vi "Continuous Swept-Sine Measurements.vi"() -> ()   [LabVIEW 2018]
doc: "Overview:\nThis VI demonstrates simultaneous frequency response, level, and distortion measurements using a discrete swept-sine technique. This example implements analog input and analog output with 'Finite Samples' sample mode which minimizes sensitivity to bandwidth issues that can cause run-time errors when performing continuous measurements. This VI also demonstrates how finite acquisitions can be read in a single large block or in a series of smaller reads.\n\nRequirements:\nLabVIEW Full Development System\nSound and Vibration Toolkit\n\nInstructions:\n1. Connect the DUT to the DSA device.\n2. Select the AO excitation channel, AI stimulus channel, and AI response channel.\n3. Run the VI.\n\nDetails:\nThis VI performs a swept sine measurement to obtain the root-mean-square (RMS) levels of the acquired stimulus and response, the frequency response of the device under test (DUT), and the harmonic distortion on the response channel. You specify the source and measurement parameters, and the swept sine VIs handle all the DAQ-specific controls required to perform the measurement. You have direct control over the source, input, averaging, and display parameters. You also specify the engineering units to use for the swept sine measurements.\n\nYou can view the time records of the acquired stimulus and response signals. From these graphs, you can see that the transition to the next test frequency always occurs at a zero crossing to minimize non-linear disturbances to the DUT. The RMS levels, frequency response, and harmonic distortion are shown on different tabs."
uses:
  <vilib>/sound2/lvsound2.llb/Sampling Mode.ctl
  <vilib>/sound2/lvsound2.llb/Sound Data Format.ctl
  <vilib>/addons/_NISVFA/_Shared subVIs/Controls/svc_Window.ctl
  <vilib>/addons/_NISVFA/_Generation/Signal Generation/SV Signal/SV Signal.lvclass/SV Signal.ctl
  <vilib>/addons/_NISVFA/_Shared subVIs/Common/svc_Get Waveform Subset (Index).vi
  <vilib>/addons/_NISVFA/_Generation/Signal Generation/SV Signal/Write Leading Synchronization Pulse Enable.vi
  <vilib>/addons/_NISVFA/_Generation/Signal Generation/SV Signal/Write Ramp-Up.vi
  <vilib>/addons/_NISVFA/_Generation/Signal Generation/SV Signal/Write Ramp-Down.vi
  <vilib>/addons/_NISVFA/_Shared subVIs/Common/svc_Get Array Subset (Index).vi
  <vilib>/addons/_NISVFA/_Shared subVIs/Common/svc_Coerce Index and Length.vi
  <vilib>/addons/_NISVFA/_Shared subVIs/Common/svc_Conditional Merge Error.vi
  <vilib>/addons/_NISVFA/_Generation/Signal Generation/SV Continuous Sweep/SV Continuous Sweep.lvclass
  C:/Program Files (x86)/National Instruments/LabVIEW 2018/vi.lib/addons/_NISVFA/_Generation/Signal Generation/SV Signal/SV Signal.lvclass
  <vilib>/addons/_NISVFA/_Generation/Signal Generation/SV Continuous Sweep/Configure Continuous Sweep.vi
  <vilib>/addons/_NISVFA/_Generation/Signal Generation/SV Signal/Write Ramp Parameters.vi
  <vilib>/addons/_NISVFA/_Generation/Signal Generation/SV Signal/Write DC Offset.vi
  <vilib>/addons/_NISVFA/_Generation/Signal Generation/SV Signal/Write Transition Profile.vi
  <vilib>/addons/_NISVFA/_Generation/Signal Generation/SV Signal/Write Pre-Measurement Settling Duration.vi
  <vilib>/addons/_NISVFA/_Generation/Signal Generation/SV Signal/Write Post-Measurement Settling Duration.vi
  <vilib>/sound2/lvsound2.llb/Sound Output Set Volume (Single).vi
  <vilib>/sound2/lvsound2.llb/Sound Output Write (DBL Single).vi
  <vilib>/sound2/lvsound2.llb/Sound Input Read (DBL).vi
  <vilib>/addons/_NISVFA/_Baseband FFT/SVFA FFT Spectrum (Complex) (1 Ch).vi
  <vilib>/addons/Sound and Vibration/svt_Single Tone Measurements/SVT Gain and Phase (Frequency).vi
  <vilib>/addons/Sound and Vibration/svt_Distortion/SVT THD and Harmonic Components (Frequency) (1 Ch).vi
  <vilib>/addons/_NISVFA/_Generation/Signal Generation/SV Signal/SV Signal.lvclass
  Program Files (x86)/National Instruments/LabVIEW 2018/examples/Sound and Vibration/SoundVib_Audio Examples.lvlib
  <vilib>/addons/Sound and Vibration/svt_Continuous Swept Sine/SoundVib_ContSweptSine.lvlib
  <vilib>/addons/Sound and Vibration/svt_Distortion/SoundVib_Distortion.lvlib
  <vilib>/addons/Sound and Vibration/svt_Single Tone Measurements/SoundVib_SingleTone.lvlib
panel:
  in  "device In":u32
  in  "device Out":u32=1
  out "Magnitude":cluster{"frequency":dbl[], "magnitude":dbl[]}(graph)
  out "Phase":cluster{"frequency":dbl[], "magnitude":dbl[]}(graph)
  out "THD":cluster{"frequency":dbl[], "THD":dbl[]}(graph)
  in  "Samples/Sec":dbl=44100.0
  in  "DC offset":dbl format="%.2f V"
  in  "amplitude":dbl=1.0 format="%.2p V"
  in  "frequency range":cluster{"start":dbl, "stop":dbl}={"start"=20000.0, "stop"=40.0} {"stop" min=0.0 format="%.2f Hz"; "start" min=0.0 format="%.2f Hz"}
  in  "duration":dbl=3.0 min=0.0 format="%.2f s"
  out "test time":u32 format="%.0f ms"
  out "error Mic":errorcluster
  out "error Spkr":errorcluster
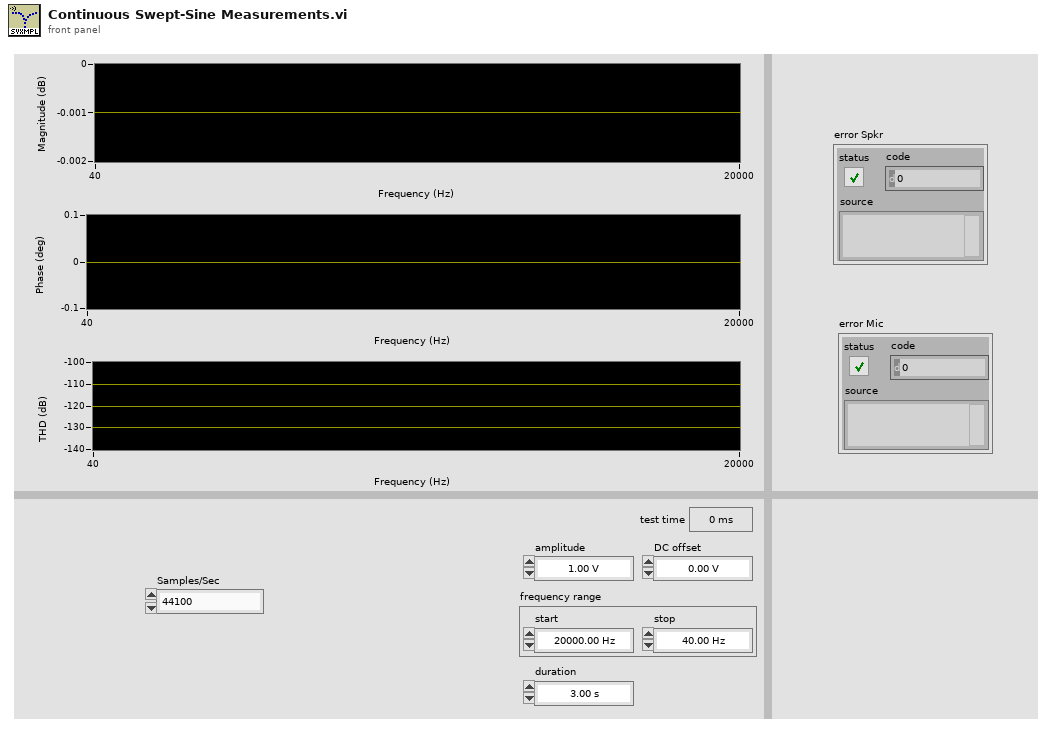
[diagram p1: front panel]
types:
  T1 = typedef "Sound Data Format.ctl" = cluster{"sample rate (S/s)":dbl, "number of channels":i32, "bits per sample":i32}
  T2 = typedef "Sampling Mode.ctl" = i32
  T3 = cluster{"start frequency":dbl, "stop frequency":dbl, "number of steps":i32}
  T4 = cluster{"profile":enum16{"Linear", "Half cosine"}, "durations [s]":cluster{"ramp-up":dbl, "transition":dbl, "ramp-down":dbl}}
  T5 = typedef "Sound Output Task ID.ctl" = u32
  T6 = typedef "Sound Input Task ID.ctl" = u32
  T7 = cluster{"averaging mode":enum16{"No averaging", "Vector averaging", "RMS averaging", "Peak hold"}, "weighting mode":enum16{"Linear", "Exponential"}, "number of averages":u32, "linear mode":enum16{"One shot", "Auto restart"}}
  T8 = typedef "svc_Window.ctl" = u32
  T9 = typedef "svc_Spectrum Info.ctl" = cluster{"channel name":string, "description":string, "x-axis units":T10, "spectral info":cluster{"spectrum type":T11, "linear/dB":enum16{"linear", "dB"}, "window":u16, "window size":i32, "FFT size":i32}, "engineering units":T12, "custom label":string, "dB reference [EU]":dbl, "peak units":enum16{"rms", "peak", "peak-peak"}, "weighting filter":T13, "spectral density?":bool, "unit label":string, "spectrum skewed?":bool, "complimentary spectrum units":T14}
  T10 = typedef "svc_X-Axis Units.ctl" = u16
  T11 = typedef "svc_Spectrum Type.ctl" = enum16{"FFT Spectrum [complex]", "Amplitude [Magnitude]", "Power [Magnitude^2]", "Cross Spectrum [complex]", "Frequency Response [Complex]"}
  T12 = typedef "svc_Engineering Units Text Ring.ctl" = u16
  T13 = typedef "svc_Weighting Filter Text Ring.ctl" = u16
  T14 = typedef "svc_Complimentary Spectrum Units.ctl" = enum16{"none", "radians", "degrees", "cycles", "imaginary"}
  T15 = cluster{"complex spectrum response":cluster{"f0":dbl, "df":dbl, "complex spectrum":cdb[]}, "spectrum info":T9}
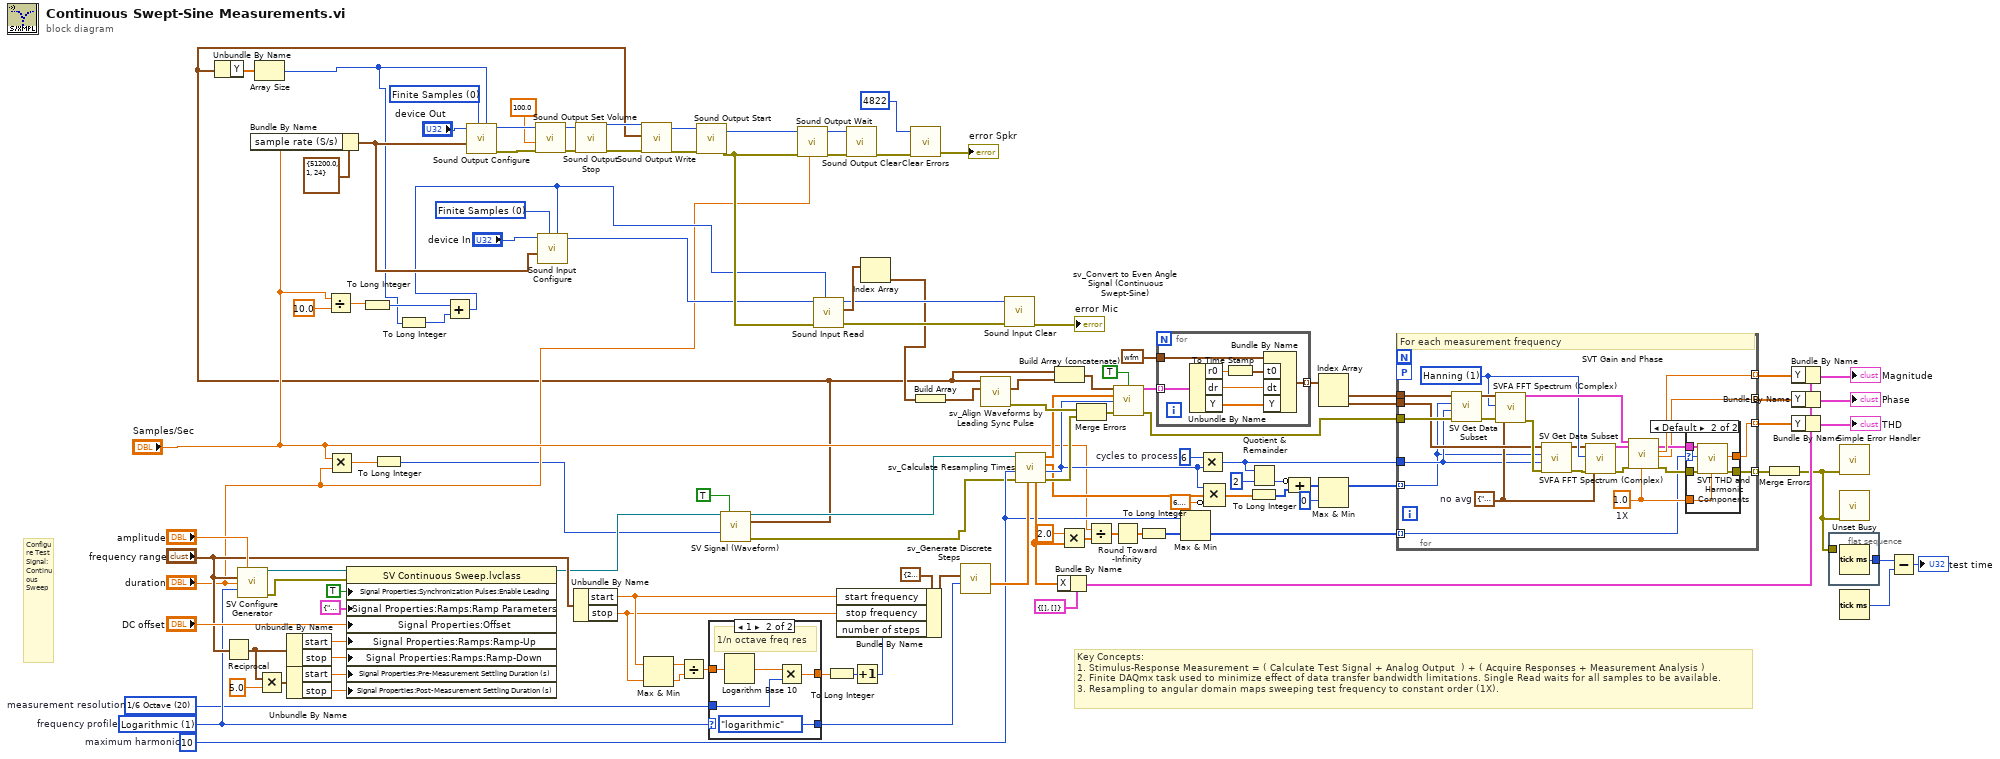
[diagram p0: block diagram]
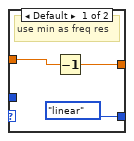
[diagram p2: hidden frame]
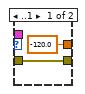
[diagram p3: hidden frame]
diagram:
  w40 = T2 0 items=["Finite Samples", "Continuous Samples"] ("sample mode")
  w42 = T2 0 items=["Finite Samples", "Continuous Samples"] ("sample mode")
  w49 = u16 20 items=["1/3 Octave"=10, "1/6 Octave"=20, "1/12 Octave"=40, "1/24 Octave"=80, "1/48 Octave"=160]  # measurement resolution
  w64 = u16 1 items=["Linear", "Logarithmic"]  # frequency profile
  w91 = 6  # cycles to process
  w52 = 10  # maximum harmonic
  # "Key Concepts:\n1. Stimulus-Response Measurement = ( Calculate Test Signal + Analog Output  ) + ( Acquire Responses + Measurement Analysis )\n2. Finite DAQmx task used to minimize effect of data transfer bandwidth limitations. Single Read waits for all samples to be available.\n3. Resampling to angular domain maps sweeping test frequency to constant order (1X)."
  # "Configure Test Signal: \nContinuous Sweep"
  n1 = Reciprocal(x="frequency range") -> (1/x=w79:cluster{"start":dbl, "stop":dbl})
  n2 = call-poly <vilib>:"SV Configure Generator.vi"("amplitude"="amplitude", "frequency range [Hz]"="frequency range", "duration [s]"="duration", "profile"=w64) -> ("signal configuration"=w119:refnum<class "SV Continuous Sweep.lvclass">, "error out"=w116:errorcluster)  [unwired: 10 in]
  n3 = Bundle By Name(cluster=T1 {"sample rate (S/s)"=51200.0, "number of channels"=1, "bits per sample"=24} ("sound format"), "sample rate (S/s)"="Samples/Sec") -> (w34:T1)
  n4 = Multiply(x=w79, y=5.0 ("stop")) -> (x*y=w80:cluster{"start":dbl, "stop":dbl})
  n5 = Unbundle By Name(w79) -> ("start"=w78:dbl, "stop"=w77:dbl)
  n6 = Unbundle By Name(w80) -> ("start"=w81:dbl, "stop"=w82:dbl)
  n7 = Divide(x="Samples/Sec", y=10.0) -> (x/y=w31:dbl)
  n8 = Multiply(x="Samples/Sec", y="duration") -> (x*y=w8:dbl)
  n9 = property class="SV Continuous Sweep.lvclass"(reference=w119, error in=w116, "Signal Properties:Synchronization Pulses:Enable Leading"=TRUE ("Synchronization Pulses:Enable Leading"), "Signal Properties:Ramps:Ramp Parameters"=T4 {"profile"=enum."Half cosine", "durations [s]"={"ramp-up"=0.01, "transition"=0.0, "ramp-down"=0.01}} ("Ramp Parameters"), "Signal Properties:Offset"="DC offset", "Signal Properties:Ramps:Ramp-Up"=w78, "Signal Properties:Ramps:Ramp-Down"=w77, "Signal Properties:Pre-Measurement Settling Duration (s)"=w81, "Signal Properties:Post-Measurement Settling Duration (s)"=w82) -> (reference out=w11:refnum<class "SV Continuous Sweep.lvclass">)  [unwired: 1 out]
  n10 = To Long Integer(number=w31) -> (32bit integer=w30:i32)
  n11 = To Long Integer(number=w8) -> (32bit integer=w7:i32)
  n12 = Unbundle By Name("frequency range") -> ("start"=w68:dbl, "stop"=w67:dbl)
  n13 = Max & Min(x=w68, y=w67) -> (max(x,y)=w73:dbl, min(x,y)=w72:dbl)
  n14 = Divide(x=w73, y=w72) -> (x/y=w71:dbl)
  n15 = case shown="1" w64 {
    tunnel: w71 -> [w121 w127]
    tunnel: [w120 w125] -> w70
    tunnel: [enum16{"linear", "logarithmic"}."linear" ("spacing") enum16{"linear", "logarithmic"}."logarithmic" ("spacing")] -> w65
    tunnel: w49 -> [_ w123]
    frame Default {
      # "use min as freq res"
      n16 = Decrement(x=w121) -> (x-1=w120:dbl)
    }
    frame 1 {
      # "1/n octave freq res"
      n17 = Logarithm Base 10(1:w127) -> (0:w126:dbl)
      n18 = Multiply(x=w126, y=w123) -> (x*y=w125:dbl)
    }
  }
  n19 = call-dynamic "SV Signal (Waveform).vi"("signal configuration"=w11, "reset"=TRUE, "samples"=w7) -> ("signal configuration"=w5:refnum<class "SV Continuous Sweep.lvclass">, "output waveform"=w3:waveform(dbl), "error out"=w4:errorcluster)  [unwired: 7 in, 3 out]
  n20 = Unbundle By Name(w3) -> ("Y"=w33:dbl[])
  n21 = Array Size(array=w33) -> (size(s)=w28:i32)
  n22 = To Long Integer(number=w28) -> (32bit integer=w29:i32)
  n23 = Add(x=w30, y=w29) -> (x+y=w18:i32)
  n24 = call <vilib>:"Sound Output Configure.vi"("number of samples/ch"=w28, "sample mode"=w42, "sound format"=w34, "device ID"="device Out") -> ("error out"=w46:errorcluster, "task ID"=w45:T5)  [unwired: 6 in]
  n25 = call-poly <vilib>:"Sound Output Set Volume.vi"("error in (no error)"=w46, "volume"=100.0, "task ID"=w45) -> ("error out"=w38:errorcluster, "task ID out"=w39:T5)  [unwired: 7 in]
  n26 = call <vilib>:"Sound Input Configure.vi"("number of samples/ch"=w18, "sample mode"=w40, "sound format"=w34, "device ID"="device In") -> ("task ID"=w17:T6)  [unwired: 6 in, 1 out]
  n27 = call <vilib>:"Sound Output Stop.vi"("error in (no error)"=w38, "task ID"=w39) -> ("error out"=w36:errorcluster, "task ID out"=w37:T5)  [unwired: 8 in]
  n28 = call-poly <vilib>:"Sound Output Write.vi"("error in (no error)"=w36, "data"=w3, "task ID"=w37) -> ("error out"=w19:errorcluster, "task ID out"=w20:T5)  [unwired: 7 in]
  n29 = call <vilib>:"Sound Output Start.vi"("error in (no error)"=w19, "task ID"=w20) -> ("error out"=w24:errorcluster, "task ID out"=w25:T5)  [unwired: 8 in]
  n30 = call <vilib>:"Sound Output Wait.vi"("timeout (sec)"="duration", "error in (no error)"=w24, "task ID"=w25) -> ("error out"=w27:errorcluster, "task ID out"=w26:T5)  [unwired: 7 in]
  n31 = call-poly <vilib>:"Sound Input Read.vi"("number of samples/ch"=w18, "error in (no error)"=w24, "task ID"=w17) -> ("error out"=w15:errorcluster, "data"=w23:waveform(dbl)[], "task ID out"=w16:T6)  [unwired: 6 in]
  n32 = To Long Integer(number=w70) -> (32bit integer=w69:i32)
  n33 = call <vilib>:"Sound Output Clear.vi"("error in (no error)"=w27, "task ID"=w26) -> ("error out"=w22:errorcluster)  [unwired: 9 in]
  n34 = Increment(x=w69) -> (x+1=w66:i32)
  n35 = Bundle By Name(cluster=T3 {"start frequency"=20.0, "stop frequency"=20000.0, "number of steps"=100} ("sweep frequencies"), "start frequency"=w68, "stop frequency"=w67, "number of steps"=w66) -> (w74:T3)
  n36 = Index Array(array=w23) -> (element=w14:waveform(dbl))  [unwired: 1 in]
  n37 = call <vilib>:"Clear Errors.vi"("error in (no error)"=w22, "specific error code to clear (0: all)"=4822) -> ("error out"=→"error Spkr":errorcluster)  [unwired: 4 in, 1 out]
  n38 = Build Array(w14) -> (w47:waveform(dbl)[])
  n39 = call <vilib>:"sv_Generate Discrete Steps.vi"("spacing"=w65, "steps"=w74) -> ("frequency list"=w60:dbl[])  [unwired: 8 in, 1 out]
  n40 = call "sv_Align Waveforms by Leading Sync Pulse.vi"("response signals"=w47, "alignment reference signal"=w3) -> ("error out"=w101:errorcluster, "aligned signals"=w2:waveform(dbl)[])  [unwired: 5 in, 3 out]
  n41 = call <vilib>:"Sound Input Clear.vi"("error in (no error)"=w15, "task ID"=w16) -> ("error out"=→"error Mic":errorcluster)  [unwired: 9 in]
  n42 = call "sv_Calculate Resampling Times.vi"("measurement frequencies in (Hz)"=w60, "error in"=w4, "maximum harmonic"=w52, "continuous sweep configuration"=w5) -> ("error out"=w100:errorcluster, "samples/rev"=w90:i32, "measurement phases (rad)"=w61:dbl[], "resampling times (s)"=w62:dbl[], "measurement frequencies (Hz)"=w53:dbl[])  [unwired: 1 in, 2 out]
  n43 = Build Array (concatenate)(w3, w2) -> (w1:waveform(dbl)[])
  n44 = Bundle By Name(cluster=cluster{"X":dbl[], "Y":dbl[]} {"X"=[], "Y"=[]} ("THD vs Amplitude"), "X"=w53) -> (w109:cluster{"X":dbl[], "Y":dbl[]})
  n45 = Multiply(x=2.0 ("y"), y=w53) -> (x*y=w57:dbl[])
  n46 = Merge Errors(w101, w100) -> (w99:errorcluster)
  n47 = Divide(x="Samples/Sec", y=w57) -> (x/y=w56:dbl[])
  n48 = Round Toward -Infinity(1:w56) -> (0:w55:dbl[])
  n49 = call <vilib>:"sv_Convert to Even Angle Signal (Continuous Swept-Sine).vi"("scaled signals [EU]"=w1, "reset? (F)"=TRUE, "new sample time [s]"=w62, "new samples/rev"=w90, "error in (no error)"=w99) -> ("even-angle signals"=w105:cluster{"r0":dbl, "dr":dbl, "Y":dbl[]}[], "error out"=w48:errorcluster)  [unwired: 6 in, 3 out]
  n50 = To Long Integer(number=w55) -> (32bit integer=w51:i32[])
  n51 = for {
    tunnel: w105 -> [w134] mode=indexing
    tunnel: waveform(dbl) {"t0"=timestamp(0 s since 1904-01-01), "dt"=1.0, "Y"=[]} ("waveform out") -> [w129]
    tunnel: [w128] -> w103 mode=indexing
    n52 = Unbundle By Name(w134) -> ("r0"=w133:dbl, "dr"=w131:dbl, "Y"=w130:dbl[])
    n53 = To Time Stamp(1:w133) -> (0:w132:timestamp)
    n54 = Bundle By Name(cluster=w129, "t0"=w132, "dt"=w131, "Y"=w130) -> (w128:waveform(dbl))
  }
  n55 = Max & Min(x=w52, y=w51) -> (min(x,y)=w50:i32[])  [unwired: 1 out]
  n56 = Multiply(x=w91, y=w90) -> (x*y=w88:i32)
  n57 = Compound Arithmetic op=MULTIPLY(w90, w61, invert 6.283185307179586) -> (w59:dbl[])
  n58 = To Long Integer(number=w59) -> (32bit integer=w87:i32[])
  n59 = Quotient & Remainder(x=w88, y=2 ("x")) -> (floor(x/y)=w89:i32)  [unwired: 1 out]
  n60 = Compound Arithmetic op=ADD(invert w89, w87) -> (w85:i32[])
  n61 = Index Array(array=w103) -> (element #1=w97:waveform(dbl), element #2=w96:waveform(dbl))  [unwired: 2 in]
  n62 = Max & Min(x=w85, y=0 ("x")) -> (max(x,y)=w84:i32[])  [unwired: 1 out]
  n63 = for {
    tunnel: w48 -> [w157]
    tunnel: [w151] -> w98 mode=indexing
    tunnel: [w150] -> w95 mode=indexing
    tunnel: w97 -> [w149]
    tunnel: w96 -> [w148]
    tunnel: [w140] -> w93 mode=indexing
    tunnel: [w139] -> w94 mode=indexing
    tunnel: w88 -> [w138]
    tunnel: w84 -> [w137] mode=indexing
    tunnel: w50 -> [w135] mode=indexing
    workers-P: _ -> [_]
    w136 = 1.0  # 1X
    w141 = T7 {"averaging mode"=enum."No averaging", "weighting mode"=enum."Exponential", "number of averages"=10, "linear mode"=enum."One shot"}  # no avg
    w152 = T8 1 items=["None"=0, "Hanning"=1, "Hamming"=2, "Blackman-Harris"=3, "Exact Blackman"=4, "Blackman"=5, "Flat Top"=6, "4 Term B-Harris "=7, "7 Term B-Harris"=8, "Low Sidelobe"=9, "Force"=64, "Exponential"=65, "Blackman Nuttall"=11, "Triangle"=30, "Bartlett-Hanning"=31, "Bohman"=32, "Parzen"=33, "Welch"=34, "Kaiser"=60, "Dolph-Chebyshev"=61, "Gaussian"=62] ("window")
    # "For each measurement frequency"
    n64 = call-poly <vilib>:"SV Get Data Subset.vi"("error in (no error)"=w157, "length (-1 = all)"=w138, "start index (0)"=w137, "waveform in"=w149) -> ("error out"=w155:errorcluster, "waveform subset"=w156:waveform(dbl))  [unwired: 2 in, 4 out]
    n65 = call-poly <vilib>:"SVFA FFT Spectrum (Complex).vi"("scaled signal [EU]"=w156, "window"=w152, "error in"=w155, "averaging parameters"=w141) -> ("complex spectrum"=w153:T15, "error out"=w154:errorcluster)  [unwired: 12 in, 2 out]
    n66 = call-poly <vilib>:"SV Get Data Subset.vi"("error in (no error)"=w154, "length (-1 = all)"=w138, "start index (0)"=w137, "waveform in"=w148) -> ("error out"=w146:errorcluster, "waveform subset"=w147:waveform(dbl))  [unwired: 2 in, 4 out]
    n67 = call-poly <vilib>:"SVFA FFT Spectrum (Complex).vi"("scaled signal [EU]"=w147, "window"=w152, "error in"=w146, "averaging parameters"=w141) -> ("complex spectrum"=w143:T15, "error out"=w142:errorcluster)  [unwired: 12 in, 2 out]
    n68 = call-poly <vilib>:"SVT Gain and Phase.vi"("complex spectrum\nstimulus X"=w153, "complex spectrum\nresponse Y"=w143, "error in (no error)"=w142, "expected fundamental frequency [Hz]"=w136) -> ("dup complex spectrum\nresponse Y"=w145:T15, "gain"=w150:dbl, "phase lag"=w139:dbl, "error out"=w144:errorcluster)  [unwired: 8 in, 4 out]
    n69 = case shown="Default" w135 {
      selector: w135 -> [_ w160]
      tunnel: [w159 w165] -> w151
      tunnel: w145 -> [_ w164]
      tunnel: w144 -> [w159 w163]
      tunnel: [-120.0 ("THD") w162] -> w140
      tunnel: w136 -> [_ w161]
      frame ..1 {
      }
      frame Default {
        n70 = call-poly <vilib>:"SVT THD and Harmonic Components.vi"("complex spectrum"=w164, "maximum harmonic"=w160, "error in (no error)"=w163, "expected fundamental frequency [Hz]"=w161) -> ("THD"=w162:dbl, "error out"=w165:errorcluster)  [unwired: 8 in, 6 out]
      }
    }
  }
  n71 = Merge Errors(w98) -> (w63:errorcluster)
  n72 = Bundle By Name(cluster=w109, "Y"=w95) -> (→"Magnitude":cluster{"X":dbl[], "Y":dbl[]})
  n73 = Bundle By Name(cluster=w109, "Y"=w94) -> (→"Phase":cluster{"X":dbl[], "Y":dbl[]})
  n74 = Bundle By Name(cluster=w109, "Y"=w93) -> (→"THD":cluster{"X":dbl[], "Y":dbl[]})
  n75 = flat-sequence {
    tunnel: [w166] -> w108
    tunnel: w63 -> [_]
    frame #0 {
      n76 = Tick Count (ms)() -> (millisecond timer value=w166:u32)
    }
  }
  n77 = call <vilib>:"Simple Error Handler.vi"("error in (no error)"=w63) -> ()  [unwired: 4 in, 5 out]
  n78 = call <vilib>:"Unset Busy.vi"("error in (no error)"=w63) -> ()  [unwired: 10 in, 1 out]
  n79 = Tick Count (ms)() -> (millisecond timer value=w106:u32)
  n80 = Subtract(x=w108, y=w106) -> (x-y=→"test time":u32)
